vi "Setup Subordinates.vi"(7 "Measurment Duration (s)":dbl, 8 "error in (no error)":errorcluster, 9 "Master Counter#":i32, 10 "Counters":T1(array[cluster]), 11 "Device Name":string) -> (0 "error out":errorcluster, 3 "Array":refnum<k21>[](array[refnum]))   [LabVIEW 2015]
uses:
  <vilib>/DAQmx/create/channels.llb/DAQmx Create Channel (CO-Pulse Generation-Time).vi
  <vilib>/DAQmx/configure/trigger.llb/DAQmx Start Trigger (Digital Edge).vi
  <vilib>/DAQmx/configure/timing.llb/DAQmx Timing (Implicit).vi
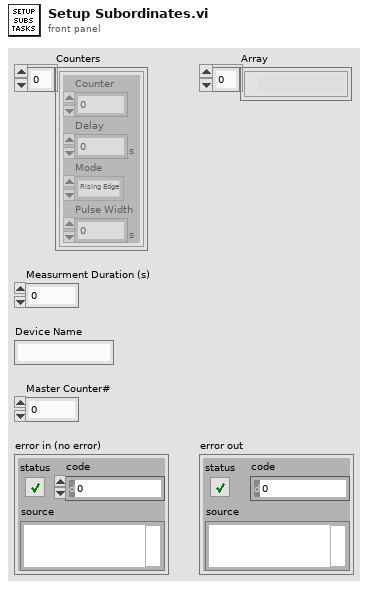
[diagram p1: front panel]
types:
  T1 = cluster{"Counter":u16, "Delay":dbl[unit], "Mode":enum16{"Rising Edge", "Falling Edge", "High Going Pulse", "Low Going Pulse"}, "Pulse Width":dbl[unit]}[]
  T2 = enum16{"Rising Edge", "Falling Edge", "High Going Pulse", "Low Going Pulse"}
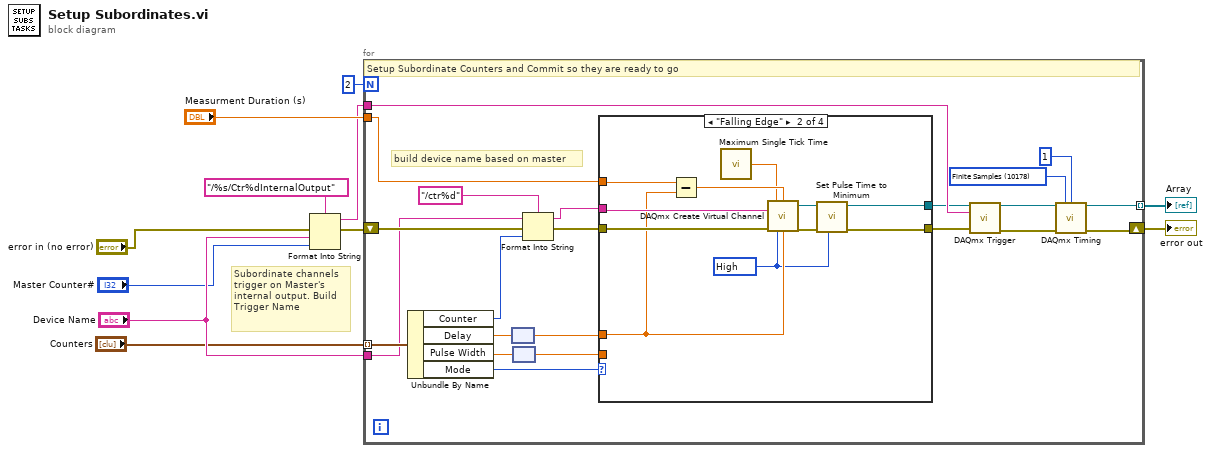
[diagram p0: block diagram]
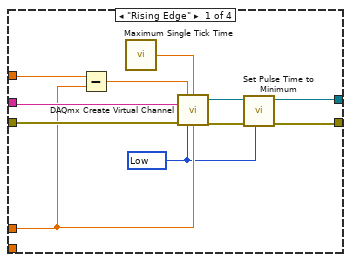
[diagram p2: hidden frame]
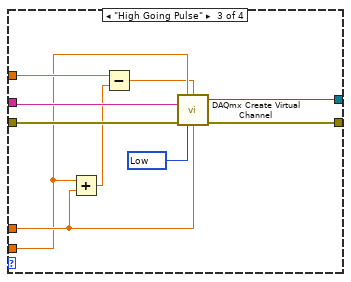
[diagram p3: hidden frame]
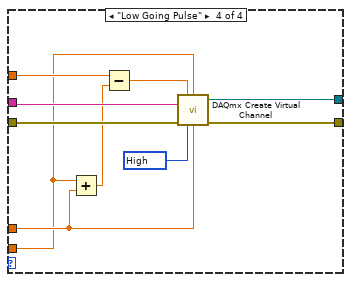
[diagram p4: hidden frame]
diagram:
  # "Subordinate channels trigger on Master's\ninternal output. Build Trigger Name"
  n1 = Format Into String(format string="/%s/Ctr%dInternalOutput", error in="error in (no error)", "Device Name", "Master Counter#") -> (resulting string=w7:string, error out=w3:errorcluster)  [unwired: 1 in]
  n2 = for {
    N: 2 -> [_]
    tunnel: "Counters" -> [w32] mode=indexing
    tunnel: "Measurment Duration (s)" -> [w13]
    shift-right: [w22] -> w8
    shift-left: w3 -> [w33]
    tunnel: "Device Name" -> [w29]
    tunnel: w7 -> [w28]
    tunnel: [w23] -> w9 mode=indexing
    w25 = 10178 items=["Finite Samples"=10178, "Continuous Samples"=10123, "Hardware Timed Single Point"=12522] ("sample mode")
    # "build device name based on master"
    # "Setup Subordinate Counters and Commit so they are ready to go"
    n3 = Unbundle By Name(w32) -> ("Counter"=w30:u16, "Delay"=w20:dbl[unit], "Pulse Width"=w19:dbl[unit], "Mode"=w12:T2)
    n4 = node(w20) -> (w18:dbl)
    n5 = node(w19) -> (w17:dbl)
    n6 = Format Into String(format string="/ctr%d", initial string=w29, error in=w33, w30) -> (resulting string=w16:string, error out=w21:errorcluster)
    n7 = case shown="\"Falling Edge\"" w12 {
      tunnel: w21 -> [w44 w55 w65 w75]
      tunnel: w18 -> [w40 w51 w59 w68]
      tunnel: w17 -> [_ _ w57 w66]
      tunnel: w16 -> [w42 w53 w61 w71]
      tunnel: [w34 w46 w64 w74] -> w15
      tunnel: [w37 w48 w63 w73] -> w14
      tunnel: w13 -> [w41 w52 w60 w70]
      frame "Rising Edge" {
        w36 = 10214 items=["High"=10192, "Low"=10214] ("idle state")
        n8 = Subtract(x=w41, y=w40) -> (x-y=w39:dbl)
        n9 = call "Maximum Single Tick Time.vi"() -> ("Maximum Single Tick (s)"=w38:dbl)
        n10 = call-poly <vilib>:"DAQmx Create Virtual Channel.vi"("high time"=w39, "low time"=w38, "counter"=w42, "error in"=w44, "idle state"=w36, "initial delay"=w40) -> ("task out"=w43:refnum<k21>, "error out"=w35:errorcluster)  [unwired: 8 in]
        n11 = call "Set Pulse Time to Minimum.vi"("Time"=w36, "error in (no error)"=w35, "Refnum in"=w43) -> ("error out"=w34:errorcluster, "Refnum out"=w37:refnum<k21>)  [unwired: 6 in, 1 out]
      }
      frame "Falling Edge" {
        w45 = 10192 items=["High"=10192, "Low"=10214] ("idle state")
        n12 = Subtract(x=w52, y=w51) -> (x-y=w50:dbl)
        n13 = call "Maximum Single Tick Time.vi"() -> ("Maximum Single Tick (s)"=w49:dbl)
        n14 = call-poly <vilib>:"DAQmx Create Virtual Channel.vi"("high time"=w49, "low time"=w50, "counter"=w53, "error in"=w55, "idle state"=w45, "initial delay"=w51) -> ("task out"=w54:refnum<k21>, "error out"=w47:errorcluster)  [unwired: 8 in]
        n15 = call "Set Pulse Time to Minimum.vi"("Time"=w45, "error in (no error)"=w47, "Refnum in"=w54) -> ("error out"=w46:errorcluster, "Refnum out"=w48:refnum<k21>)  [unwired: 6 in, 1 out]
      }
      frame "High Going Pulse" {
        w62 = 10214 items=["High"=10192, "Low"=10214] ("idle state")
        n16 = Add(x=w57, y=w59) -> (x+y=w58:dbl)
        n17 = Subtract(x=w60, y=w58) -> (x-y=w56:dbl)
        n18 = call-poly <vilib>:"DAQmx Create Virtual Channel.vi"("high time"=w57, "low time"=w56, "counter"=w61, "error in"=w65, "idle state"=w62, "initial delay"=w59) -> ("task out"=w63:refnum<k21>, "error out"=w64:errorcluster)  [unwired: 8 in]
      }
      frame "Low Going Pulse" {
        w72 = 10192 items=["High"=10192, "Low"=10214] ("idle state")
        n19 = Add(x=w66, y=w68) -> (x+y=w67:dbl)
        n20 = Subtract(x=w70, y=w67) -> (x-y=w69:dbl)
        n21 = call-poly <vilib>:"DAQmx Create Virtual Channel.vi"("high time"=w69, "low time"=w66, "counter"=w71, "error in"=w75, "idle state"=w72, "initial delay"=w68) -> ("task out"=w73:refnum<k21>, "error out"=w74:errorcluster)  [unwired: 8 in]
      }
    }
    n22 = call-poly <vilib>:"DAQmx Trigger.vi"("task/channels in"=w14, "source"=w28, "error in"=w15) -> ("task out"=w27:refnum<k21>, "error out"=w26:errorcluster)  [unwired: 11 in]
    n23 = call-poly <vilib>:"DAQmx Timing.vi"("task/channels in"=w27, "sample mode"=w25, "samples per channel"=1, "error in"=w26) -> ("task out"=w23:refnum<k21>, "error out"=w22:errorcluster)  [unwired: 10 in]
  }
  "Array" <- w9
  "error out" <- w8
